vi "GOOP_IconOCR.vi"(9 "BackColor(T), TextColor(F)":bool, 10 "BackColor Or TextColor(8bit)":u8, 11 "Icon":u8[][](array[numeric])) -> (3 "String":string)   [LabVIEW 2020]
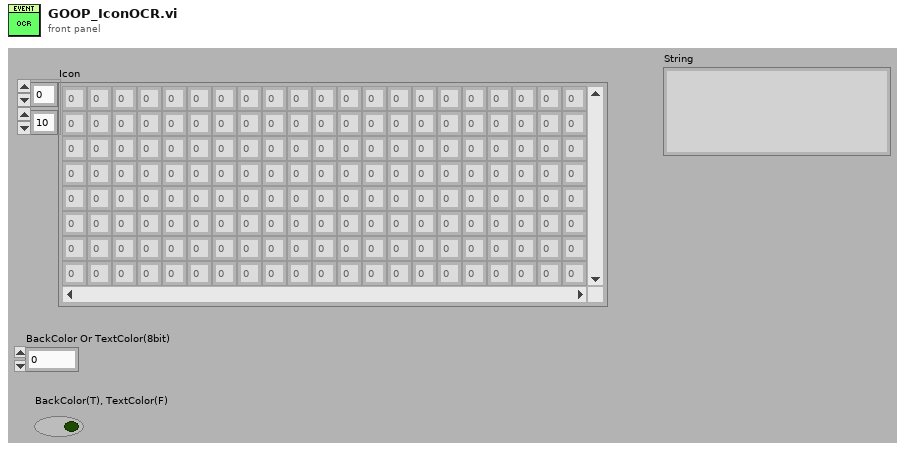
[diagram p1: front panel]
types:
  T1 = cluster{"Character":string, cluster{"Char":bool[][]}[]}
  T2 = cluster{"Character":string, cluster{"Char":bool[][]}[]}[]
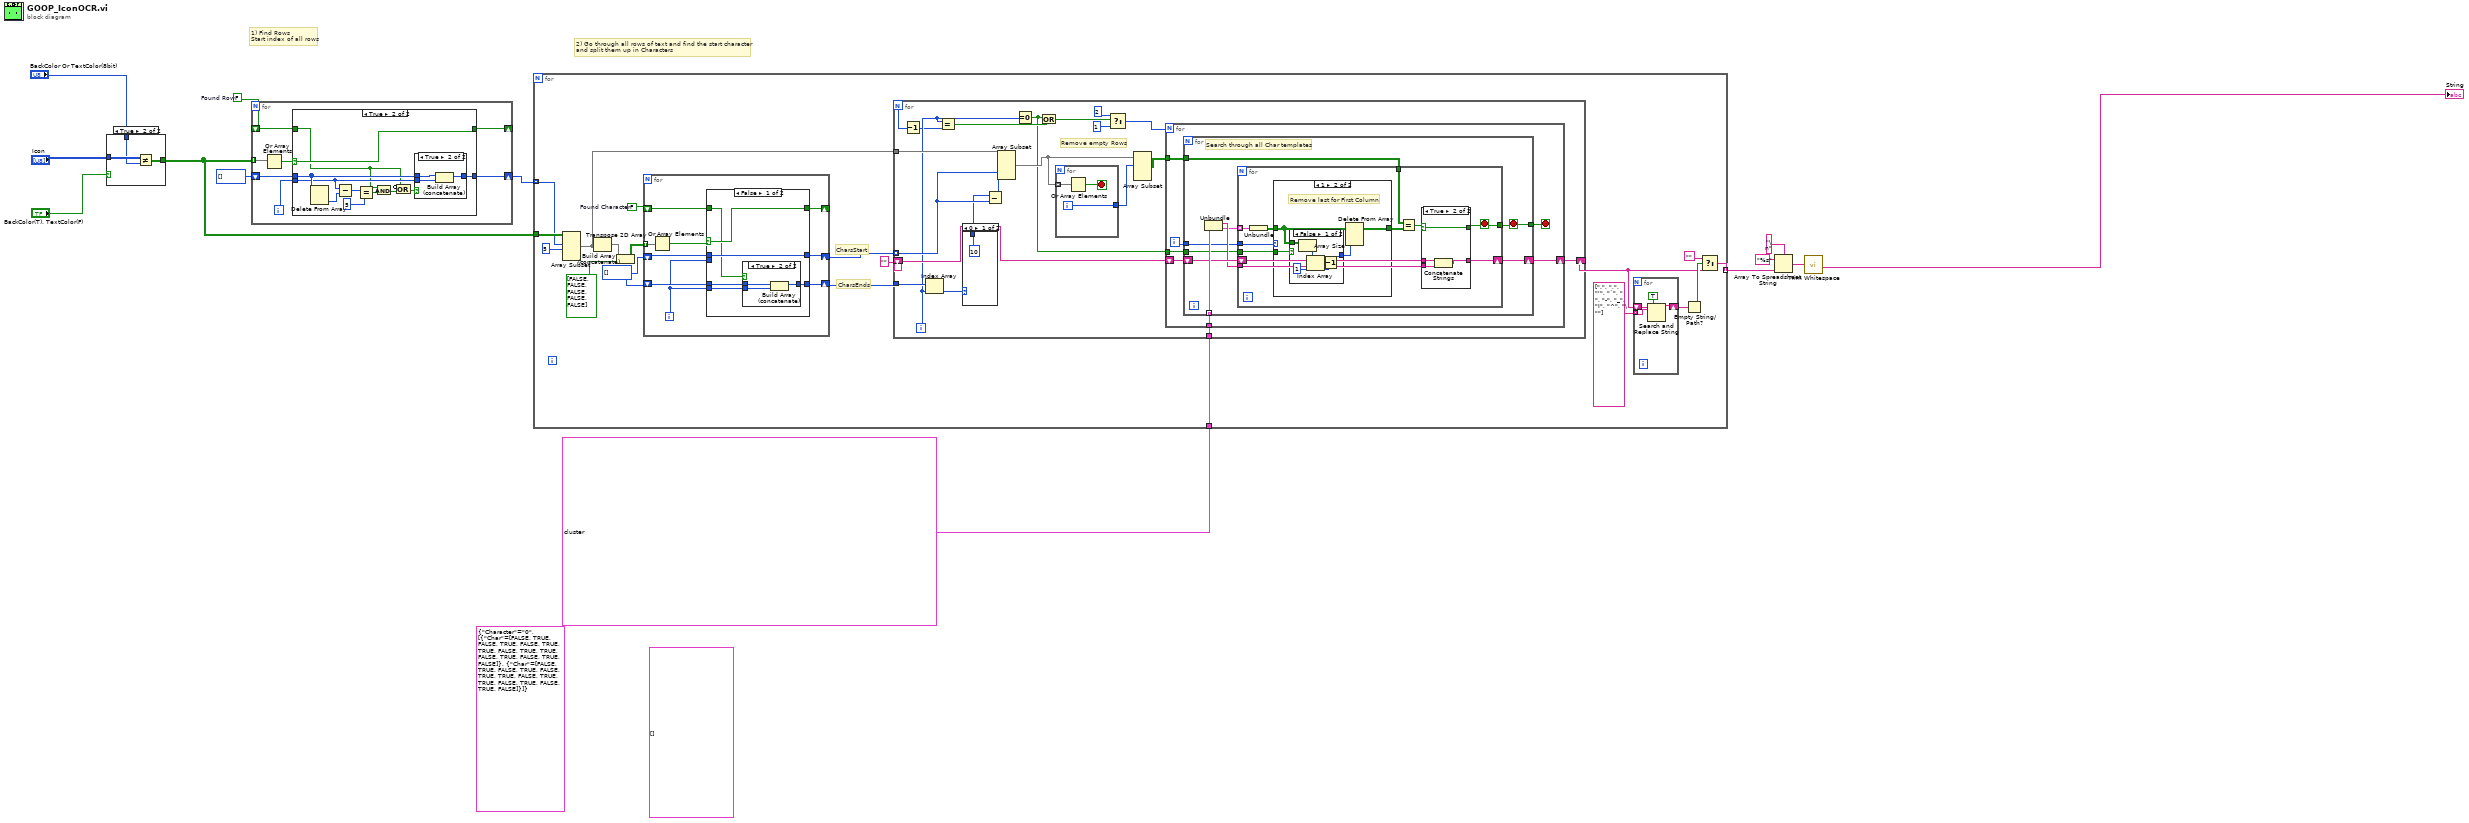
[diagram p0: block diagram]
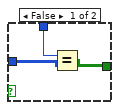
[diagram p2: hidden frame]
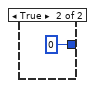
[diagram p4: hidden frame]
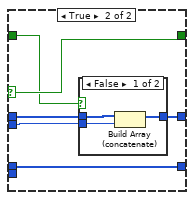
[diagram p8: hidden frame]
diagram:
  (unwired) cluster{"Char":bool[][]}[] []
  (unwired) T1 {"Character"="0", [{"Char"=[[FALSE, TRUE, FALSE], [TRUE, FALSE, TRUE], [TRUE, FALSE, TRUE], [TRUE, FALSE, TRUE], [FALSE, TRUE, FALSE]]}, {"Char"=[[FALSE, TRUE, FALSE], [TRUE, FALSE, TRUE], [TRUE, FALSE, TRUE], [TRUE, FALSE, TRUE], [FALSE, TRUE, FALSE]]}]}
  w9 = FALSE  # Found Row
  # "2) Go through all rows of text and find the start character\nand split them up in Characters"
  # "1) Find Rows\nStart index of all rows"
  n1 = case shown="True" "BackColor(T), TextColor(F)" {
    tunnel: [w14 w19] -> w12
    tunnel: "Icon" -> [w16 w18]
    tunnel: "BackColor Or TextColor(8bit)" -> [w15 w17]
    frame False {
      n2 = Equal?(x=w15, y=w16) -> (x = y?=w14:bool[][])
    }
    frame True {
      n3 = Not Equal?(x=w18, y=w17) -> (x != y?=w19:bool[][])
    }
  }
  n4 = for {
    tunnel: w12 -> [w26] mode=indexing
    shift-right: [w23] -> _
    shift-left: w9 -> [w24]
    shift-right: [w21] -> w7
    shift-left: i32[] [] -> [w22]
    i -> [w20]
    n5 = Or Array Elements(Boolean array=w26) -> (logical OR=w25:bool)
    n6 = case shown="True" w25 {
      selector: w25 -> [w28 w39]
      tunnel: w24 -> [_ w30]
      tunnel: [w28 w39] -> w23
      tunnel: w22 -> [w27 w37]
      tunnel: [w27 w38] -> w21
      tunnel: w20 -> [_ w36]
      frame False {
      }
      frame True {
        n7 = Delete From Array(array=w37) -> (deleted portion=w35:i32)  [unwired: 2 in, 1 out]
        n8 = Subtract(x=w36, y=w35) -> (x-y=w34:i32)
        n9 = Equal?(x=w34, y=5) -> (x = y?=w32:bool)
        n10 = And(x=w30, y=w32) -> (x .and. y?=w31:bool)
        n11 = Compound Arithmetic op=OR(invert w30, w31) -> (w29:bool)
        n12 = case shown="True" w29 {
          tunnel: w37 -> [w40 w43]
          tunnel: [w40 w42] -> w38
          tunnel: w36 -> [_ w41]
          frame False {
          }
          frame True {
            n13 = Build Array (concatenate)(w43, w41) -> (w42:i32[])
          }
        }
      }
    }
  }
  n14 = for {
    tunnel: w7 -> [w61] mode=indexing
    tunnel: w12 -> [w62]
    tunnel: T2 data[9401B] ("Array") -> [w56]
    tunnel: [w48] -> w6 mode=indexing
    w55 = i32[] []
    w59 = FALSE  # Found Character
    # "CharsEnds"
    # "CharsStart"
    n15 = Array Subset(array=w62, index (row)=w61, length (row)=5 ("length")) -> (w58:bool[][])  [unwired: 2 in]
    n16 = Transpose 2D Array(2D array=w58) -> (transposed array=w46:bool[][])
    n17 = Build Array (concatenate)(w46, bool[] [FALSE, FALSE, FALSE, FALSE, FALSE] ("array")) -> (w45:bool[][])
    n18 = for {
      tunnel: w45 -> [w144] mode=indexing
      shift-right: [w143] -> _
      shift-left: w59 -> [w142]
      shift-right: [w140] -> w57
      shift-left: w55 -> [w139]
      shift-right: [w137] -> w54
      shift-left: w55 -> [w138]
      i -> [w136]
      n19 = Or Array Elements(Boolean array=w144) -> (logical OR=w141:bool)
      n20 = case shown="False" w141 {
        selector: w141 -> [w150 w160]
        tunnel: w142 -> [w148 w156]
        tunnel: [w150 w160] -> w143
        tunnel: w139 -> [w149 w159]
        tunnel: [w149 w158] -> w140
        tunnel: w136 -> [_ w157]
        tunnel: w138 -> [w147 w155]
        tunnel: [w146 w155] -> w137
        tunnel: w136 -> [w145 _]
        frame False {
          n21 = case shown="True" w148 {
            tunnel: w147 -> [w151 w154]
            tunnel: [w151 w153] -> w146
            tunnel: w145 -> [_ w152]
            frame False {
            }
            frame True {
              n22 = Build Array (concatenate)(w154, w152) -> (w153:i32[])
            }
          }
        }
        frame True {
          n23 = case shown="False" w156 {
            tunnel: w159 -> [w163 w164]
            tunnel: [w162 w164] -> w158
            tunnel: w157 -> [w161 _]
            frame False {
              n24 = Build Array (concatenate)(w163, w161) -> (w162:i32[])
            }
            frame True {
            }
          }
        }
      }
    }
    n25 = for {
      N -> [w71]
      tunnel: w58 -> [w87]
      tunnel: w57 -> [w78] mode=indexing
      tunnel: w56 -> [w86]
      tunnel: w54 -> [w82]
      shift-right: [w79] -> w49
      shift-left: "" -> [w80]
      i -> [w70]
      # "Remove empty Rows"
      n26 = Decrement(x=w71) -> (x-1=w67:i32)
      n27 = Index Array(array=w82, index=w70) -> (element=w81:i32)
      n28 = Equal?(x=w70, y=w67) -> (x = y?=w69:bool)
      n29 = case shown="0" w81 {
        selector: w81 -> [_ w135]
        tunnel: [10 w135] -> w76
        frame 0 {
        }
        frame Default {
        }
      }
      n30 = Subtract(x=w76, y=w78) -> (x-y=w77:i32)
      n31 = Array Subset(array=w87, index (col)=w78, length (col)=w77) -> (w85:bool[][])  [unwired: 2 in]
      n32 = Equal To 0?(x=w70) -> (x = 0?=w68:bool)
      n33 = Or(x=w68, y=w69) -> (x .or. y?=w75:bool)
      n34 = for {
        tunnel: w85 -> [w133] mode=indexing
        tunnel: [w131] -> w84
        i -> [w131]
        stop <- w132 stop-if-true
        n35 = Or Array Elements(Boolean array=w133) -> (logical OR=w132:bool)
      }
      n36 = Select(t=2, s=w75, f=1) -> (s? t:f=w73:i32)
      n37 = Array Subset(array=w85, index (row)=w84) -> (w83:bool[][])  [unwired: 3 in]
      n38 = for {
        N: w73 -> [_]
        tunnel: w86 -> [w94]
        tunnel: w83 -> [w93]
        shift-right: [w91] -> w79
        shift-left: w80 -> [w92]
        tunnel: w68 -> [w88]
        i -> [w89]
        stop <- w90 stop-if-true
        n39 = for {
          tunnel: w94 -> [w103] mode=indexing
          tunnel: w93 -> [w96]
          shift-right: [w100] -> w91
          shift-left: w92 -> [w102]
          tunnel: [w98] -> w90
          tunnel: w89 -> [w97]
          tunnel: w88 -> [w95]
          stop <- w98 stop-if-true
          # "Search through all Char templates"
          n40 = Unbundle(w103) -> ("Character"=w101:string, w99:cluster{"Char":bool[][]}[])
          n41 = for {
            tunnel: w101 -> [w113]
            tunnel: w96 -> [w111]
            tunnel: w99 -> [w110] mode=indexing
            tunnel: [w108] -> w98
            shift-right: [w112] -> w100
            shift-left: w102 -> [w114]
            tunnel: w97 -> [w107]
            tunnel: w95 -> [w104]
            stop <- w108 stop-if-true
            n42 = Unbundle(w110) -> ("Char"=w106:bool[][])
            n43 = case shown="1" w107 {
              tunnel: w106 -> [w115 w116]
              tunnel: [w115 w118] -> w105
              tunnel: w104 -> [_ w117]
              frame 0, Default {
              }
              frame 1 {
                # "Remove last for First Column"
                n44 = case shown="False" w117 {
                  tunnel: [w120 0 ("disabled index (col)")] -> w119
                  tunnel: w116 -> [w124 _]
                  frame False {
                    n45 = Array Size(array=w124) -> (size(s)=w123:i32[])
                    n46 = Index Array(array=w123, index=1) -> (element=w121:i32)
                    n47 = Decrement(x=w121) -> (x-1=w120:i32)
                  }
                  frame True {
                  }
                }
                n48 = Delete From Array(array=w116, index (col)=w119) -> (array with subset deleted=w118:bool[][])  [unwired: 2 in, 1 out]
              }
            }
            n49 = Equal?(x=w111, y=w105) -> (x = y?=w109:bool)
            n50 = case shown="True" w109 {
              selector: w109 -> [_ w127]
              tunnel: w114 -> [w126 w130]
              tunnel: [w126 w129] -> w112
              tunnel: w113 -> [_ w128]
              tunnel: [_ w127] -> w108
              frame False {
              }
              frame True {
                n51 = Concatenate Strings(w130, w128) -> (w129:string)
              }
            }
          }
        }
      }
    }
    n52 = for {
      shift-right: [w65] -> w51
      shift-left: w49 -> [w66]
      tunnel: string[] [".", ",", "'", "`", " ", "-", "_", "I", "^", "\""] -> [w63] mode=indexing
      n53 = Search and Replace String(replace all?=TRUE ("replace all? (F)"), input string=w66, search string=w63) -> (result string=w65:string)  [unwired: 5 in, 3 out]
    }
    n54 = Empty String/Path?(string/path=w51) -> (empty?=w50:bool)
    n55 = Select(t="", s=w50, f=w49) -> (s? t:f=w48:string)
  }
  n56 = Array To Spreadsheet String(delimiter (Tab)="\n", array=w6, 3:"%s" ("format string")) -> (spreadsheet string=w3:string)
  n57 = call <vilib>:"Trim Whitespace.vi"("string"=w3) -> ("trimmed string"=→"String":string)  [unwired: 1 in]
